vi "Main.vi"(11 "Module Admin":refnum<class "Delacor_lib_QMH_Module Admin.lvclass">) -> ()   [LabVIEW 2019, in "Modulo_Singleton_WHL.lvlib"]
doc: "This template is based off of the Queued Message Handler design pattern and the Queued Message Handler project template that ships with LabVIEW.\n\nThe main difference is that the queue is private to this module and communication between modules is performed via Broadcast and Request events.\n\nRequest events are wrapped in public API methods and are handled in the Event Handling Loop (EHL) of this VI. Any module can register for Broadcast events sent by this module. The EHL generates messages based on user interface actions.\n\nThe Message Handling Loop (MHL) processes messages generated by the EHL, or by other messages. The messages are string values, so new messages can be added easily to the Message Cases case structure in the MHL. Each message cluster can also provide an optional value for Message Data, which is a variant that can be converted to whatever message-specific data is required.\n_____\nBased on Delacor QMH Project Template 5.0.0.82."
uses:
  Modulo_Singleton_WHL.lvlib
  <vilib>/Delacor/Delacor QMH/Libraries/Module Admin_class/Delacor_lib_QMH_Module Admin.lvclass
  Module Data--cluster.ctl
  Stop helper loop Argument--cluster.ctl
  <vilib>/Delacor/Delacor QMH/Libraries/Message Queue_class/Delacor_lib_QMH_Message Queue.lvclass/Delacor_lib_QMH_Message Queue.ctl
  Stop Argument--cluster.ctl
  <vilib>/Delacor/Delacor QMH/Libraries/Module Admin_class/Delacor_lib_QMH_Module Admin.lvclass/Delacor_lib_QMH_Module Admin.ctl
  <vilib>/Utility/miscctls.llb/LVPointTypeDef.ctl
  <vilib>/Delacor/Delacor QMH/Libraries/Message Queue_class/Delacor_lib_QMH_Enqueue Message (Single).vi
  <vilib>/Delacor/Delacor QMH/Libraries/Module Admin_class/Delacor_lib_QMH_Get External Launch.vi
  <vilib>/Utility/error.llb/Error Cluster From Error Code.vi
  <vilib>/ErrorRing/Error Ring.xnode
  <vilib>/Delacor/Delacor QMH/Libraries/Message Queue_class/Delacor_lib_QMH_Message Queue.lvclass
panel:
  out "Time Stamp":timestamp
  in  "Simulate MHL Error":bool
  in  "Simulate EHL Error":bool
  out "error out":errorcluster
  out "Status":string
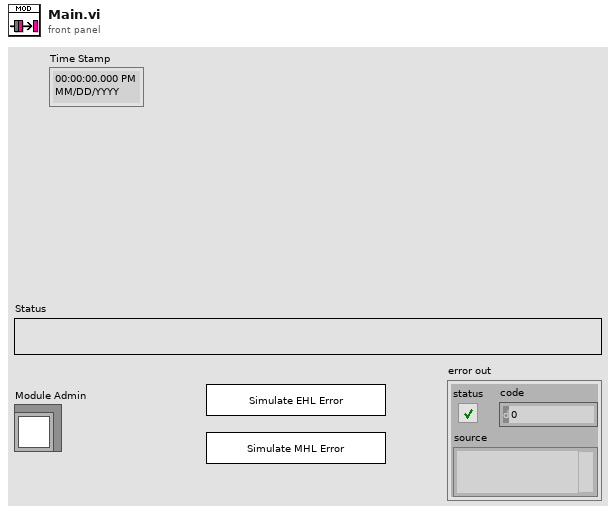
[diagram p1: front panel]
types:
  T1 = typedef "Modulo_Singleton_WHL.lvlib/Request Events--cluster.ctl" = cluster{"Stop Module":refnum<user-event>, "Show Panel":refnum<user-event>, "Hide Panel":refnum<user-event>, "Get Module Execution Status":refnum<user-event>, "Show Diagram":refnum<user-event>, "Start helper loop":refnum<user-event>, "Stop helper loop":refnum<user-event>}
  T2 = typedef "Modulo_Singleton_WHL.lvlib/Module Data--cluster.ctl" = cluster{"Status":string}
  T3 = typedef "Modulo_Singleton_WHL.lvlib/Stop helper loop Argument--cluster.ctl" = cluster{"Boolean":bool}
  T4 = enum32{"invalid lock state", "Not Locked", "Locked (No Password)", "Password-protected"}
  T5 = typedef "Modulo_Singleton_WHL.lvlib/Stop Argument--cluster.ctl" = cluster{"Origin":string, "Exit via Stop Module Req?":bool, "Wait for Module to stop?":bool}
  T6 = typedef "LVPointTypeDef.ctl" = cluster{"Horizontal":i16, "Vertical":i16}
  T7 = enum32{"Invalid", "Standard", "Closed", "Hidden", "Minimized", "Maximized"}
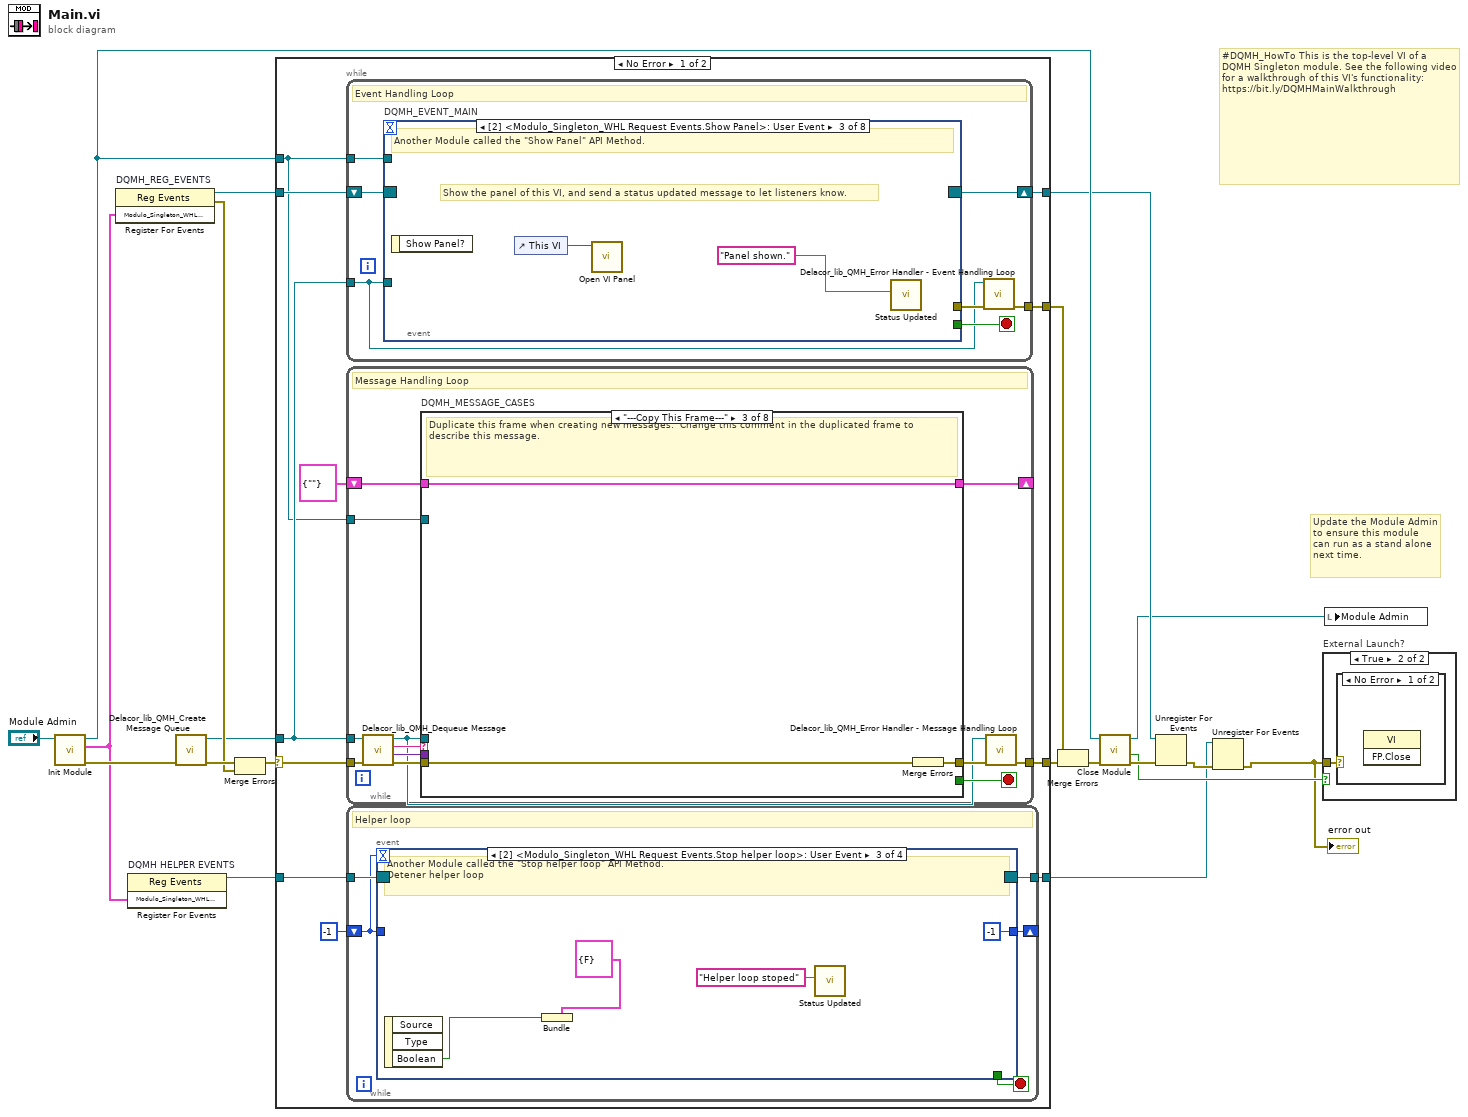
[diagram p0: block diagram]
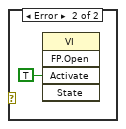
[diagram p3: hidden frame]
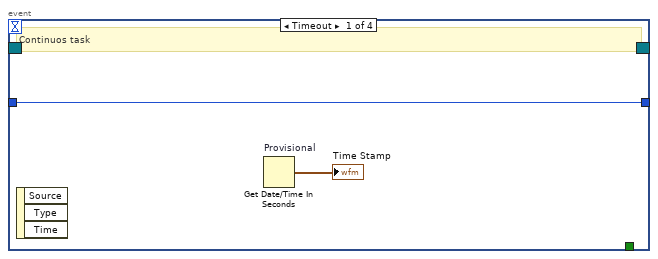
[diagram p4: hidden frame]
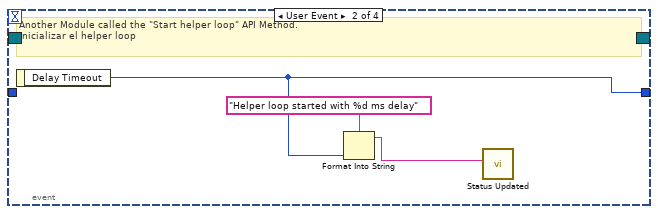
[diagram p5: hidden frame]
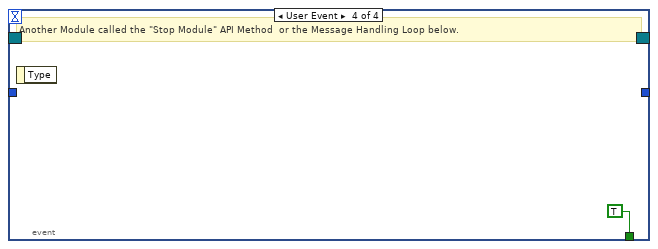
[diagram p6: hidden frame]
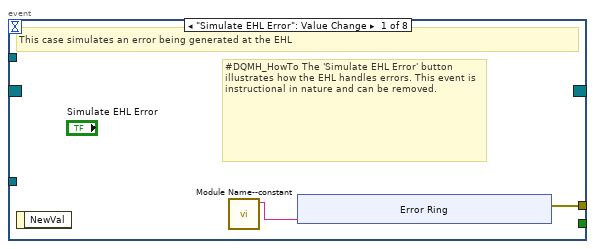
[diagram p7: hidden frame]
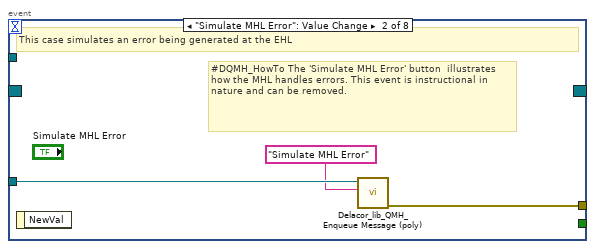
[diagram p8: hidden frame]
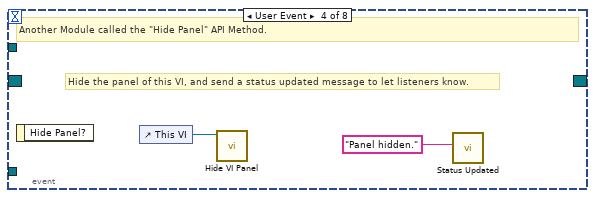
[diagram p9: hidden frame]
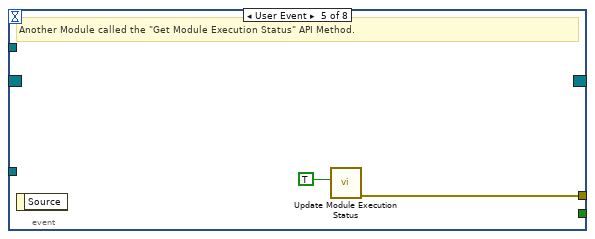
[diagram p10: hidden frame]
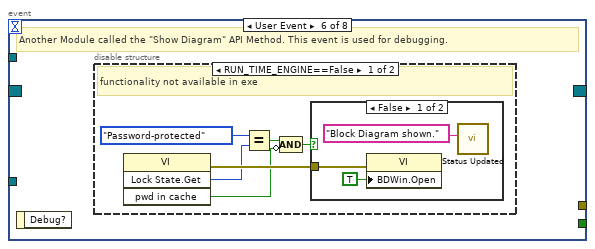
[diagram p11: hidden frame]
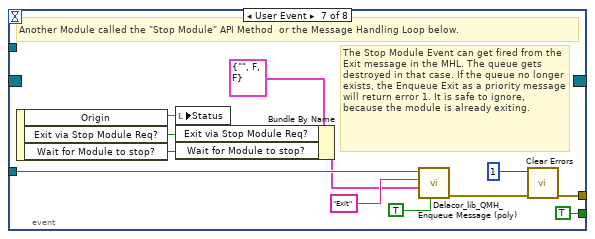
[diagram p14: hidden frame]
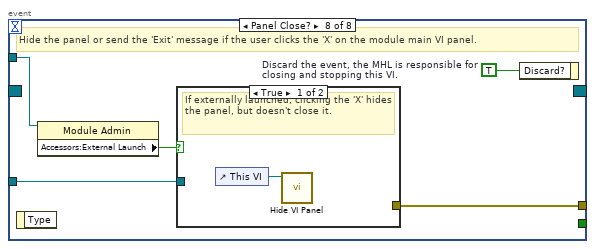
[diagram p15: hidden frame]
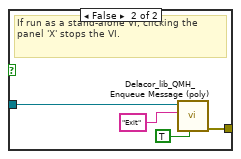
[diagram p16: hidden frame]
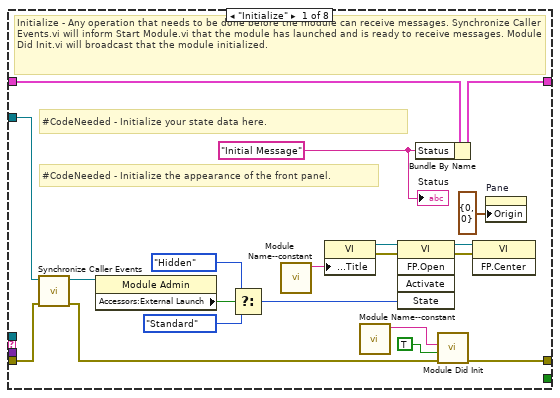
[diagram p17: hidden frame]
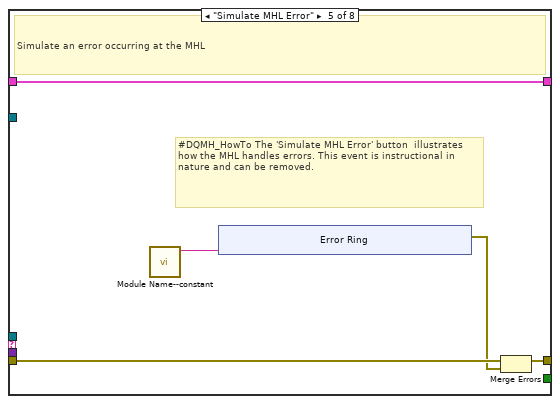
[diagram p20: hidden frame]
diagram:
  # "#DQMH_HowTo This is the top-level VI of a DQMH Singleton module. See the following video for a walkthrough of this VI's functionality: https://bit.ly/DQMHMainWalkthrough"
  # "Update the Module Admin to ensure this module can run as a stand alone next time."
  n1 = call "Init Module.vi"("Singleton Module Admin in"="Module Admin") -> ("error out"=w19:errorcluster, "Modulo_Singleton_WHL Request Events"=w4:T1, "Singleton Module Admin out"=w12:refnum<class "Delacor_lib_QMH_Module Admin.lvclass">)  [unwired: 8 in]
  n2 = register-events "DQMH_REG_EVENTS"(w4) -> (reference out=w10:refnum<event-registration>, error out=w13:errorcluster)  [unwired: 2 in]
  n3 = register-events "DQMH HELPER EVENTS"(w4) -> (reference out=w5:refnum<event-registration>)  [unwired: 2 in, 1 out]
  n4 = call <vilib>:"Delacor_lib_QMH_Create Message Queue.vi"("error in (no error)"=w19) -> ("error out"=w15:errorcluster, "Message Queue"=w9:refnum<class "Delacor_lib_QMH_Message Queue.lvclass">)  [unwired: 9 in]
  n5 = Merge Errors(w15, w13) -> (w14:errorcluster)
  n6 = case shown="No Error" w14 {
    selector: w14 -> [w29 w203]
    tunnel: [w31 w202] -> w20
    tunnel: [w28 w208] -> w11
    tunnel: w10 -> [w26 w208]
    tunnel: w9 -> [w25 w201]
    tunnel: [w30 _] -> w17
    tunnel: w12 -> [w24 w204]
    tunnel: w5 -> [w23 w200]
    tunnel: [w22 w200] -> w1
    frame No Error {
      n7 = while {
        tunnel: w25 -> [w47]
        shift-right: [w50] -> w28
        shift-left: w26 -> [w51]
        tunnel: [w52] -> w30
        tunnel: w24 -> [w48]
        stop <- w49 stop-if-true
        # "Event Handling Loop"
        n8 = event "DQMH_EVENT_MAIN" shown="[2] <Modulo_Singleton_WHL Request Events.Show Panel>: User Event" {
          selector: w51 -> [_ _ _ _ _ _ _ _]
          dyn-events: [_ _ _ _ _ _ _ _] -> w50
          timeout: _ -> [_ _ _ _ _ _ _ _]
          tunnel: [_ _ _ _ _ _ TRUE ("Discard?") _] -> w49
          tunnel: w47 -> [_ w64 _ _ _ _ w88 w95]
          tunnel: [w55 w65 _ _ w71 _ w91 w97] -> w53
          tunnel: w48 -> [_ _ _ _ _ _ _ w94]
          event "Simulate EHL Error": Value Change {
            # "#DQMH_HowTo The 'Simulate EHL Error' button  illustrates how the EHL handles errors. This event is instructional in nature and can be removed."
            # "This case simulates an error being generated at the EHL"
            n9 = event-data() -> ()  [unwired: 1 in, 1 out]
            n10 = call "Module Name--constant.vi"() -> ("Module Name"=w54:string)  [unwired: 11 in]
            n11 = xnode "Error Ring"("parameter 0"=w54) -> ("error out"=w55:errorcluster)
          }
          event "Simulate MHL Error": Value Change {
            # "#DQMH_HowTo The 'Simulate MHL Error' button  illustrates how the MHL handles errors. This event is instructional in nature and can be removed."
            # "This case simulates an error being generated at the EHL"
            n12 = event-data() -> ()  [unwired: 1 in, 1 out]
            n13 = call-poly <vilib>:"Delacor_lib_QMH_Enqueue Message (poly).vi"("Message"="Simulate MHL Error", "Message Queue in"=w64) -> ("error out"=w65:errorcluster)  [unwired: 8 in, 1 out]
          }
          event User Event {
            # "Show the panel of this VI, and send a status updated message to let listeners know."
            # "Another Module called the \"Show Panel\" API Method."
            n14 = event-data() -> ()  [unwired: 1 in, 1 out]
            n15 = control-ref of="This VI"() -> (w67:refnum<vi>)
            n16 = call "Open VI Panel.vi"("VI"=w67) -> ()  [unwired: 10 in, 1 out]
            n17 = call "Status Updated.vi"("Status"="Panel shown." ("format string")) -> ()  [unwired: 10 in, 1 out]
          }
          event User Event {
            # "Hide the panel of this VI, and send a status updated message to let listeners know."
            # "Another Module called the \"Hide Panel\" API Method."
            n18 = event-data() -> ()  [unwired: 1 in, 1 out]
            n19 = control-ref of="This VI"() -> (w69:refnum<vi>)
            n20 = call "Hide VI Panel.vi"("VI"=w69) -> ()  [unwired: 10 in, 1 out]
            n21 = call "Status Updated.vi"("Status"="Panel hidden." ("format string")) -> ()  [unwired: 10 in, 1 out]
          }
          event User Event {
            # "Another Module called the \"Get Module Execution Status\" API Method."
            n22 = event-data() -> ()  [unwired: 1 in, 1 out]
            n23 = call "Update Module Execution Status.vi"("Running?"=TRUE) -> ("error out"=w71:errorcluster)  [unwired: 10 in]
          }
          event User Event {
            # "Another Module called the \"Show Diagram\" API Method. This event is used for debugging."
            n24 = event-data() -> ()  [unwired: 1 in, 1 out]
            n25 = disable-structure shown="RUN_TIME_ENGINE==False" {
              frame condition #0 (active) {
                # "functionality not available in exe"
                n26 = invoke class="VI" method="Lock State.Get"() -> (error out=w77:errorcluster, "Get Lock State"=w76:T4, "pwd in cache"=w73:bool)  [unwired: 4 in, 1 out]
                n27 = Equal?(x=T4."Password-protected", y=w76) -> (x = y?=w74:bool)
                n28 = Compound Arithmetic op=AND(w74, invert w73) -> (w72:bool)
                n29 = case shown="False" w72 {
                  tunnel: w77 -> [w80 _]
                  frame False {
                    n30 = property class="VI"(error in=w80, "BDWin.Open"=TRUE ("Block Diagram Window:Open")) -> ()  [unwired: 1 in, 2 out]
                    n31 = call "Status Updated.vi"("Status"="Block Diagram shown." ("format string")) -> ()  [unwired: 10 in, 1 out]
                  }
                  frame True {
                    # "Password-protected VI, and the password is not in the cache. Do not show the diagram."
                  }
                }
              }
              frame condition #1 {
              }
            }
          }
          event User Event {
            # "The Stop Module Event can get fired from the Exit message in the MHL. The queue gets destroyed in that case. If the queue no longer exists, the Enqueue Exit as a priority message will return error 1. It is safe to ignore, because the module is already exiting."
            # "Another Module called the \"Stop Module\" API Method  or the Message Handling Loop below."
            n32 = event-data() -> ("Origin"=w87:string, "Exit via Stop Module Req?"=w83:bool, "Wait for Module to stop?"=w82:bool)  [unwired: 1 in]
            n33 = local write "Status"(w87) -> ()
            n34 = Bundle By Name(cluster=T5 {"Origin"="", "Exit via Stop Module Req?"=FALSE, "Wait for Module to stop?"=FALSE} ("Stop Argument"), "Exit via Stop Module Req?"=w83, "Wait for Module to stop?"=w82) -> (w81:T5)
            n35 = call-poly <vilib>:"Delacor_lib_QMH_Enqueue Message (poly).vi"("Priority Message? (F)"=TRUE, "Message Data"=w81, "Message"="Exit", "Message Queue in"=w88) -> ("error out"=w92:errorcluster)  [unwired: 6 in, 1 out]
            n36 = call <vilib>:"Clear Errors.vi"("error in (no error)"=w92, "specific error code to clear (0: all)"=1) -> ("error out"=w91:errorcluster)  [unwired: 4 in, 1 out]
          }
          event Panel Close? {
            w96 = TRUE  # Discard the event, the MHL is responsible for closing and stopping this VI.
            # "Hide the panel or send the 'Exit' message if the user clicks the 'X' on the module main VI panel."
            n37 = event-data() -> ()  [unwired: 1 in, 1 out]
            n38 = property class="Module Admin"(reference=w94) -> ("Accessors:External Launch"=w93:bool)  [unwired: 1 in, 2 out]
            n39 = case shown="True" w93 {
              tunnel: w95 -> [_ w101]
              tunnel: [_ w102] -> w97
              frame True {
                # "If externally launched, clicking the 'X' hides the panel, but doesn't close it."
                n40 = control-ref of="This VI"() -> (w98:refnum<vi>)
                n41 = call "Hide VI Panel.vi"("VI"=w98) -> ()  [unwired: 10 in, 1 out]
              }
              frame False {
                # "If run as a stand-alone VI, clicking the panel 'X' stops the VI."
                n42 = call-poly <vilib>:"Delacor_lib_QMH_Enqueue Message (poly).vi"("Priority Message? (F)"=TRUE, "Message"="Exit", "Message Queue in"=w101) -> ("error out"=w102:errorcluster)  [unwired: 7 in, 1 out]
              }
            }
            n43 = event-data("Discard?"=w96) -> ()  [unwired: 1 in, 1 out]
          }
        }
        n44 = call-dynamic "Delacor_lib_QMH_Error Handler - Event Handling Loop.vi"("error in (no error)"=w53, "Message Queue in"=w47) -> ("dup error in"=w52:errorcluster)  [unwired: 8 in, 1 out]
      }
      n45 = while {
        tunnel: w25 -> [w105]
        shift-right: [w109] -> _
        shift-left: T2 {"Status"=""} ("Data Cluster") -> [w110]
        tunnel: w29 -> [w113]
        tunnel: [w111] -> w31
        tunnel: w24 -> [w103]
        stop <- w108 stop-if-true
        # "Message Handling Loop"
        n46 = call-dynamic "Delacor_lib_QMH_Dequeue Message.vi"("error in (no error)"=w113, "Message Queue in"=w105) -> ("error out"=w112:errorcluster, "Message Data"=w106:variant, "Message"=w107:string, "Message Queue out"=w104:refnum<class "Delacor_lib_QMH_Message Queue.lvclass">)  [unwired: 6 in]
        n47 = case "DQMH_MESSAGE_CASES" shown="\"---Copy This Frame---\"" w107 {
          selector: w107 -> [_ _ _ _ _ _ _ w187]
          tunnel: w104 -> [_ _ _ _ _ w157 w179 _]
          tunnel: w112 -> [w132 w136 w139 w141 w146 w164 w185 w189]
          tunnel: [w130 w136 w138 w141 w145 w160 w182 w190] -> w114
          tunnel: w110 -> [w121 w135 w137 w140 w143 w159 w178 w188]
          tunnel: [w120 w135 w137 w140 w143 w159 w178 w188] -> w109
          tunnel: [_ _ _ _ _ _ w177 _] -> w108
          tunnel: w106 -> [_ _ _ _ _ w158 w176 _]
          tunnel: w103 -> [w122 _ _ _ _ w156 w171 _]
          frame "Initialize" {
            w115 = "Initial Message" ("Initial Message")
            # "#CodeNeeded - Initialize the appearance of the front panel."
            # "#CodeNeeded - Initialize your state data here."
            # "Initialize - Any operation that needs to be done before the module can receive messages. Synchronize Caller Events.vi will inform Start Module.vi that the module has launched and is ready to receive messages. Module Did Init.vi will broadcast that the module initialized."
            n48 = call "Synchronize Caller Events.vi"("error in (no error)"=w132, "Singleton Module Admin in"=w122) -> ("error out"=w131:errorcluster, "Singleton Module Admin out"=w117:refnum<class "Delacor_lib_QMH_Module Admin.lvclass">)  [unwired: 8 in]
            n49 = property class="Module Admin"(reference=w117) -> ("Accessors:External Launch"=w126:bool)  [unwired: 1 in, 2 out]
            n50 = Select(t=T7."Hidden" ("State"), s=w126, f=T7."Standard" ("State")) -> (s? t:f=w123:T7)
            n51 = call "Module Name--constant.vi"() -> ("Module Name"=w129:string)  [unwired: 11 in]
            n52 = property class="VI"("Front Panel.Title"=w129) -> (reference out=w128:refnum<vi>, error out=w134:errorcluster)  [unwired: 2 in]
            n53 = call "Module Name--constant.vi"() -> ("Module Name"=w118:string)  [unwired: 11 in]
            n54 = invoke class="VI" method="FP.Open"(reference=w128, error in=w134, "State"=w123) -> (reference out=w127:refnum<vi>, error out=w133:errorcluster)  [unwired: 2 in, 3 out]
            n55 = Bundle By Name(cluster=w121, "Status"=w115) -> (w120:T2)
            n56 = call "Module Did Init.vi"("error in (no error)"=w131, "Initialized?"=TRUE, "Origin"=w118) -> ("error out"=w130:errorcluster)  [unwired: 8 in]
            n57 = invoke class="VI" method="FP.Center"(reference=w127, error in=w133) -> ()  [unwired: 1 in, 3 out]
            n58 = property on="Pane" class="Pane"("Origin"=T6 {"Horizontal"=0, "Vertical"=0}) -> ()  [unwired: 2 in, 2 out]
            "Status" <- w115
          }
          frame "--- Module Specific ---" {
            # "Separator -- The following cases handle messages specific to this Module."
          }
          frame "---Copy This Frame---" {
            # "Duplicate this frame when creating new messages.  Change this comment in the duplicated frame to describe this message."
            n59 = Merge Errors(w139) -> (w138:errorcluster)
          }
          frame "--- Exit and Error Handling---" {
            # "Separator - The following cases handle errors and exit messages."
          }
          frame "Simulate MHL Error" {
            # "#DQMH_HowTo The 'Simulate MHL Error' button  illustrates how the MHL handles errors. This event is instructional in nature and can be removed."
            # "Simulate an error occurring at the MHL"
            n60 = call "Module Name--constant.vi"() -> ("Module Name"=w142:string)  [unwired: 11 in]
            n61 = xnode "Error Ring"("parameter 0"=w142) -> ("error out"=w144:errorcluster)
            n62 = Merge Errors(w146, w144) -> (w145:errorcluster)
          }
          frame "Error" {
            # "#CodeRecommended - If you ever change the name of this \"Error\" message, you'll need to update the name in the Check Loop Error.vi as well."
            # "#CodeRecommended - If the module is running in standalone mode (External Launch = FALSE), this code will pop up an error dialog and call the 'Exit' message if an error occurs. Add more fine-grained error handling here."
            # "Error - Check the error message data and respond accordingly. This message is sent by the \"Error Handler\" VIs at the end of each loop in this application."
            n63 = property class="Module Admin"(reference=w156) -> ("Accessors:External Launch"=w155:bool)  [unwired: 1 in, 2 out]
            n64 = Variant To Data(error in=w164, type=errorcluster {"status"=FALSE, "code"=0, "source"=""} ("error constant"), Variant=w158) -> (data=w165:errorcluster, error out=w162:errorcluster)
            n65 = call "Module Name--constant.vi"() -> ("Module Name"=w154:string)  [unwired: 11 in]
            n66 = call "Error Reported.vi"("Additional Information"=w154, "Error"=w165) -> ()  [unwired: 9 in, 1 out]
            n67 = case shown="False" w155 {
              tunnel: [w170 _] -> w161
              tunnel: w157 -> [w168 _]
              tunnel: w165 -> [w169 _]
              frame False {
                # "If the module is running standalone, then pop up an error dialog and call the \"Exit\" message."
                n68 = call <vilib>:"Simple Error Handler.vi"("error in (no error)"=w169) -> ()  [unwired: 4 in, 5 out]
                n69 = call-poly <vilib>:"Delacor_lib_QMH_Enqueue Message (poly).vi"("Priority Message? (F)"=TRUE, "Message"="Exit", "Message Queue in"=w168) -> ("error out"=w170:errorcluster)  [unwired: 7 in, 1 out]
              }
              frame True {
                # "If the module was launched externally, calling the Error Reported broadcast VI is the only action performed by the \"Error\" message. The module's caller can then process the error appropriately."
              }
            }
            n70 = Merge Errors(w162, w161) -> (w160:errorcluster)
            n71 = local write "error out"(w160) -> ()
          }
          frame "Exit" {
            w175 = 91  # 91: not all Exit messages will have an argument
            w177 = TRUE  # Stop the VI
            # "Release the message queue reference"
            # "#CodeNeeded - Add any required cleanup code here"
            # "Exit - Exit the application."
            n72 = Variant To Data(error in=w185, type=T5 {"Origin"="", "Exit via Stop Module Req?"=FALSE, "Wait for Module to stop?"=FALSE} ("Stop Argument"), Variant=w176) -> (data=w173:T5, error out=w181:errorcluster)
            n73 = call <vilib>:"Clear Errors.vi"("error in (no error)"=w181, "specific error code to clear (0: all)"=w175) -> ("error out"=w184:errorcluster)  [unwired: 4 in, 1 out]
            n74 = control-ref of="This VI"() -> (w172:refnum<vi>)
            n75 = call-dynamic "Delacor_lib_QMH_Release Message Queue.vi"("error in (no error)"=w184, "Message Queue"=w179) -> ("error out"=w183:errorcluster)  [unwired: 9 in]
            n76 = call "Handle Exit.vi"("Stop Argument"=w173, "Admin in"=w171, "VI reference"=w172) -> ("error out"=w180:errorcluster)  [unwired: 7 in, 1 out]
            n77 = Merge Errors(w183, w180) -> (w182:errorcluster)
          }
          frame Default {
            # "'Default' case only runs if there is a message that isn't defined in any of the other cases.  Output a programming error."
            n78 = call "Module Name--constant.vi"() -> ("Module Name"=w186:string)  [unwired: 11 in]
            n79 = xnode "Error Ring"("parameter 0"=w187, "parameter 1"=w186) -> ("error out"=w191:errorcluster)
            n80 = Merge Errors(w189, w191) -> (w190:errorcluster)
          }
        }
        n81 = call-dynamic "Delacor_lib_QMH_Error Handler - Message Handling Loop.vi"("error in (no error)"=w114, "Message Queue in"=w104) -> ("dup error in"=w111:errorcluster)  [unwired: 8 in, 1 out]
      }
      n82 = while {
        tunnel: w23 -> [w36]
        tunnel: [w35] -> w22
        shift-right: [w33] -> _
        shift-left: -1 -> [w32]
        stop <- w34 stop-if-true
        # "Helper loop"
        n83 = event shown="[2] <Modulo_Singleton_WHL Request Events.Stop helper loop>: User Event" {
          selector: w36 -> [_ _ _ _]
          dyn-events: [_ _ _ _] -> w35
          timeout: w32 -> [_ _ _ _]
          tunnel: [_ _ _ TRUE] -> w34
          tunnel: [w38 w41 -1 _] -> w33
          tunnel: w32 -> [w38 _ _ _]
          event Timeout {
            # "Continuos task"
            n84 = event-data() -> ()  [unwired: 1 in, 3 out]
            n85 = Get Date/Time In Seconds "Provisional"() -> (seconds since 1Jan1904=→"Time Stamp":timestamp)
          }
          event User Event {
            # "Another Module called the \"Start helper loop\" API Method.\nInicializar el helper loop"
            n86 = event-data() -> ("Delay Timeout"=w41:i32)  [unwired: 1 in]
            n87 = Format Into String(format string="Helper loop started with %d ms delay", w41) -> (resulting string=w39:string)  [unwired: 2 in, 1 out]
            n88 = call "Status Updated.vi"("Status"=w39) -> ()  [unwired: 10 in, 1 out]
          }
          event User Event {
            # "Another Module called the \"Stop helper loop\" API Method.\nDetener helper loop"
            n89 = event-data() -> ("Boolean"=w44:bool)  [unwired: 1 in, 2 out]
            n90 = Bundle(cluster=T3 {"Boolean"=FALSE} ("Stop helper loop Argument"), "Boolean"=w44) -> ()  [unwired: 1 out]
            n91 = call "Status Updated.vi"("Status"="Helper loop stoped") -> ()  [unwired: 10 in, 1 out]
          }
          event User Event {
            # "Another Module called the \"Stop Module\" API Method  or the Message Handling Loop below."
            n92 = event-data() -> ()  [unwired: 1 in, 1 out]
          }
        }
      }
    }
    frame Error {
      # "Synchronize Caller Events.vi will inform Start Module.vi that the module has launched and will let the code calling Start Module.vi register for broadcasts and would permit the caller receive the broadcast that an error occurred at launch time."
      n93 = call-dynamic "Delacor_lib_QMH_Release Message Queue.vi"("error in (no error)"=w203, "Message Queue"=w201) -> ("error out"=w202:errorcluster)  [unwired: 9 in]
      n94 = call "Synchronize Caller Events.vi"("Singleton Module Admin in"=w204) -> ("error out"=w209:errorcluster)  [unwired: 9 in, 1 out]
      n95 = call "Module Name--constant.vi"() -> ("Module Name"=w207:string)  [unwired: 11 in]
      n96 = Format Into String(format string="An error occurred during initialization. %s is no longer running.", w207) -> (resulting string=w205:string)  [unwired: 2 in, 1 out]
      n97 = Merge Errors(w202, w209) -> (w210:errorcluster)
      n98 = call "Error Reported.vi"("Additional Information"=w205, "Error"=w210) -> ()  [unwired: 9 in, 1 out]
    }
  }
  n99 = Merge Errors(w17, w20) -> (w16:errorcluster)
  n100 = call "Close Module.vi"("error in (no error)"=w16, "Module Admin in"=w12) -> ("error out"=w18:errorcluster, "External Launch"=w6:bool, "Module Admin out"=w7:refnum<class "Delacor_lib_QMH_Module Admin.lvclass">)  [unwired: 7 in]
  n101 = Unregister For Events(event registration refnum=w11, error in=w18) -> (error out=w3:errorcluster)
  n102 = Unregister For Events(event registration refnum=w1, error in=w3) -> (error out=w2:errorcluster)
  "error out" <- w2
  n103 = case "External Launch?" shown="True" w6 {
    tunnel: w2 -> [_ w211]
    frame False {
    }
    frame True {
      n104 = case shown="No Error" w211 {
        frame No Error {
          n105 = invoke class="VI" method="FP.Close"() -> ()  [unwired: 3 in, 3 out]
        }
        frame Error {
          n106 = invoke class="VI" method="FP.Open"("Activate"=TRUE ("Activate?")) -> ()  [unwired: 4 in, 5 out]
        }
      }
    }
  }
  n107 = local write "Module Admin"(w7) -> ()
